vi "LVObject to JSON - Aggregate Descendant - Returns JSON Object With Descendant JSON Object.vi"() -> ()   [LabVIEW 2017, in "Tests.lvlib"]
uses:
  Tests.lvlib
  Flatten To JSON Object/Flatten To JSON Object.lvclass
  Temperature Forecast/Temperature Forecast.lvclass
  C:/Users/de200256/Code/logmanoriginal/jsontext-object-serialization/Tests/Weather Forecast/Weather Forecast.lvclass
  <vilib>/addons/_JKI Toolkits/Caraya/classes/Assert/Assert Equal Value_Variant.vi
  <vilib>/addons/_JKI Toolkits/Caraya/classes/Test/Test.lvclass
  <vilib>/addons/_JKI Toolkits/Caraya/classes/Assert/Assert.lvclass
  City/City.lvclass
panel:
  out "error out":errorcluster
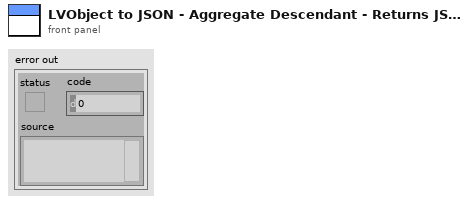
[diagram p1: front panel]
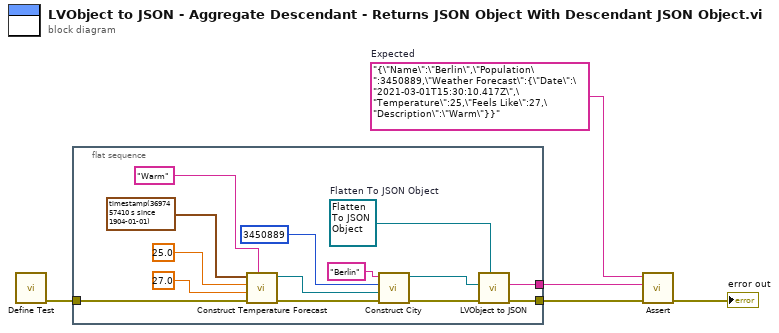
[diagram p0: block diagram]
diagram:
  w1 = "{\"Name\":\"Berlin\",\"Population\":3450889,\"Weather Forecast\":{\"Date\":\"2021-03-01T15:30:10.417Z\",\"Temperature\":25,\"Feels Like\":27,\"Description\":\"Warm\"}}"  # Expected
  n1 = call <vilib>:"Define Test.vi"() -> ("error out"=w4:errorcluster)  [unwired: 11 in]
  n2 = flat-sequence {
    tunnel: w4 -> [w14]
    tunnel: [w18] -> w3
    tunnel: [w17] -> w2
    frame #0 {
      w19 = refnum<class "Flatten To JSON Object.lvclass"> refnum  # Flatten To JSON Object
      n3 = call "Construct Temperature Forecast.vi"("Description"="Warm", "error in (no error)"=w14, "Feels Like [°C]"=27.0, "Temperature [°C]"=25.0, "Date"=timestamp(3697457410.417 s since 1904-01-01)) -> ("error out"=w13:errorcluster, "Temperature Forecast"=w12:refnum<class "Temperature Forecast.lvclass">)  [unwired: 5 in]
      n4 = call "Construct City.vi"("error in (no error)"=w13, "Weather Forecast"=w12, "Population"=u32 3450889, "Name"="Berlin") -> ("error out"=w16:errorcluster, "City"=w15:refnum<class "City.lvclass">)  [unwired: 6 in]
      n5 = call-dynamic "LVObject to JSON.vi"("Flatten To JSON Object in"=w19, "error in (no error)"=w16, "Object"=w15) -> ("error out"=w18:errorcluster, "<JSON>Object"=w17:string)  [unwired: 7 in]
    }
  }
  n6 = call-poly <vilib>:"Assert.vi"("error in (no error)"=w3, "Y"=w2, "X"=w1) -> ("error out"=→"error out":errorcluster)  [unwired: 8 in]
